vi "escribeGaugeVolt_AVG.vi"(1 "Vin":sgl) -> (0 "V_V out":cluster{"Max":sgl, "Vin":sgl, "Min":sgl})   [LabVIEW 2018]
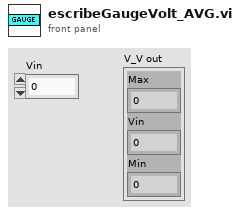
[diagram p1: front panel]
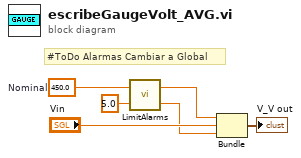
[diagram p0: block diagram]
diagram:
  w2 = sgl 450.0  # Nominal
  # "#ToDo Alarmas Cambiar a Global"
  n1 = call "LimitAlarms.vi"("Value"=sgl 5.0, "Parameter"=w2) -> ("Min"=w5:sgl, "Max"=w4:sgl)
  n2 = Bundle("Max"=w4, "Vin"="Vin", "Min"=w5) -> (→"V_V out":cluster{"Max":sgl, "Vin":sgl, "Min":sgl})  [unwired: 1 in]
